vi "DAQ.vi"(8 "data":bool[](array[boolean]), 11 "lines":tag) -> ()   [LabVIEW 2016]
uses:
  <vilib>/DAQmx/write.llb/DAQmx Write (Digital 1D Bool 1Chan 1Samp).vi
  <vilib>/DAQmx/create/channels.llb/DAQmx Create Channel (DO-Digital Output).vi
  <vilib>/DAQmx/miscellaneous.llb/DAQmx Fill In Error Info.vi
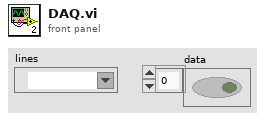
[diagram p1: front panel]
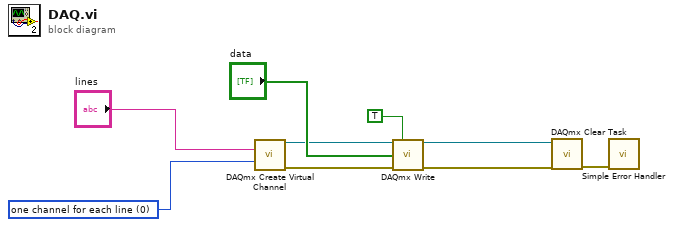
[diagram p0: block diagram]
diagram:
  w2 = 0 items=["one channel for each line", "one channel for all lines"] ("line grouping")
  n1 = call-poly <vilib>:"DAQmx Create Virtual Channel.vi"("lines"="lines", "line grouping"=w2) -> ("task out"=w3:refnum<k21>, "error out"=w4:errorcluster)  [unwired: 12 in]
  n2 = call-poly <vilib>:"DAQmx Write.vi"("task/channels in"=w3, "auto start"=TRUE, "data"="data", "error in"=w4) -> ("task out"=w5:refnum<k21>, "error out"=w6:errorcluster)  [unwired: 9 in, 1 out]
  n3 = call <vilib>:"DAQmx Clear Task.vi"("task in"=w5, "error in"=w6) -> ("error out"=w7:errorcluster)  [unwired: 13 in]
  n4 = call <vilib>:"Simple Error Handler.vi"("error in (no error)"=w7) -> ()  [unwired: 4 in, 5 out]
